vi "MainPicMotV1.vi"() -> ()   [LabVIEW 2010]
uses:
  <vilib>/Instr/_visa.llb/VISA Flush IO Buffer Mask.ctl
  Variable globale 1.vi
  <vilib>/Instr/_visa.llb/VISA Configure Serial Port (Instr).vi
panel:
  out "Iteration 3":i32
  out "Iteration reception":i32
  out "Iteration Envoi":i32
  out "Checksum calculé":i32
  out "Checksum reçu":i32
  out "Data":i32
  out "Type de donnee (ID)":i32
  out "Byte Start ?":bool
  out "Retour 2":string
  in  "Donnee":i32=138 min=0 max=255
  in  "Type":i32=138 min=138 max=139
  in  "stop secu":bool
  in  "STOP":bool
  out "error out":errorcluster caption="sortie d'erreur"
  in  "baud rate (9600)":u32=9600 caption="débit en bauds (9600)"
  in  "Port Com":refnum<visa-resource-name> caption="Nom de ressource VISA"
  # "Envoi"
  # "Réception"
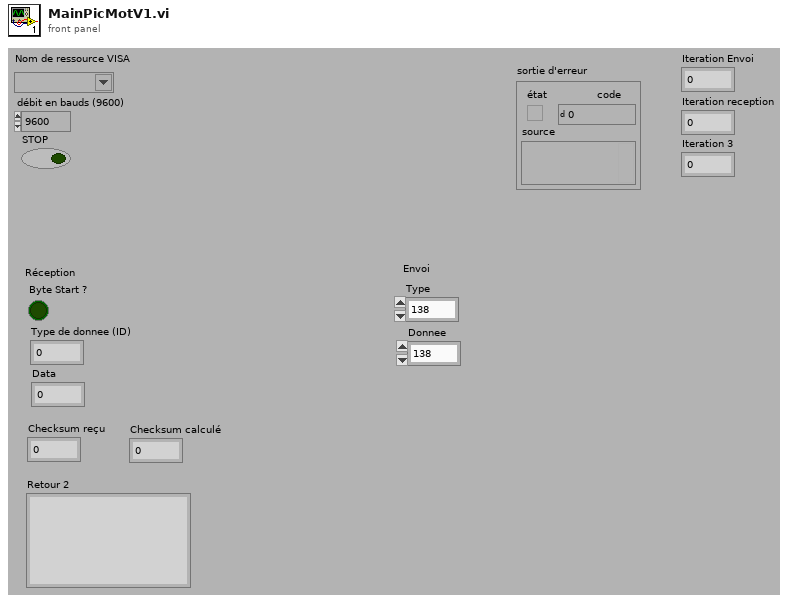
[diagram p1: front panel]
types:
  T1 = typedef "VISA Flush IO Buffer Mask.ctl" = u16
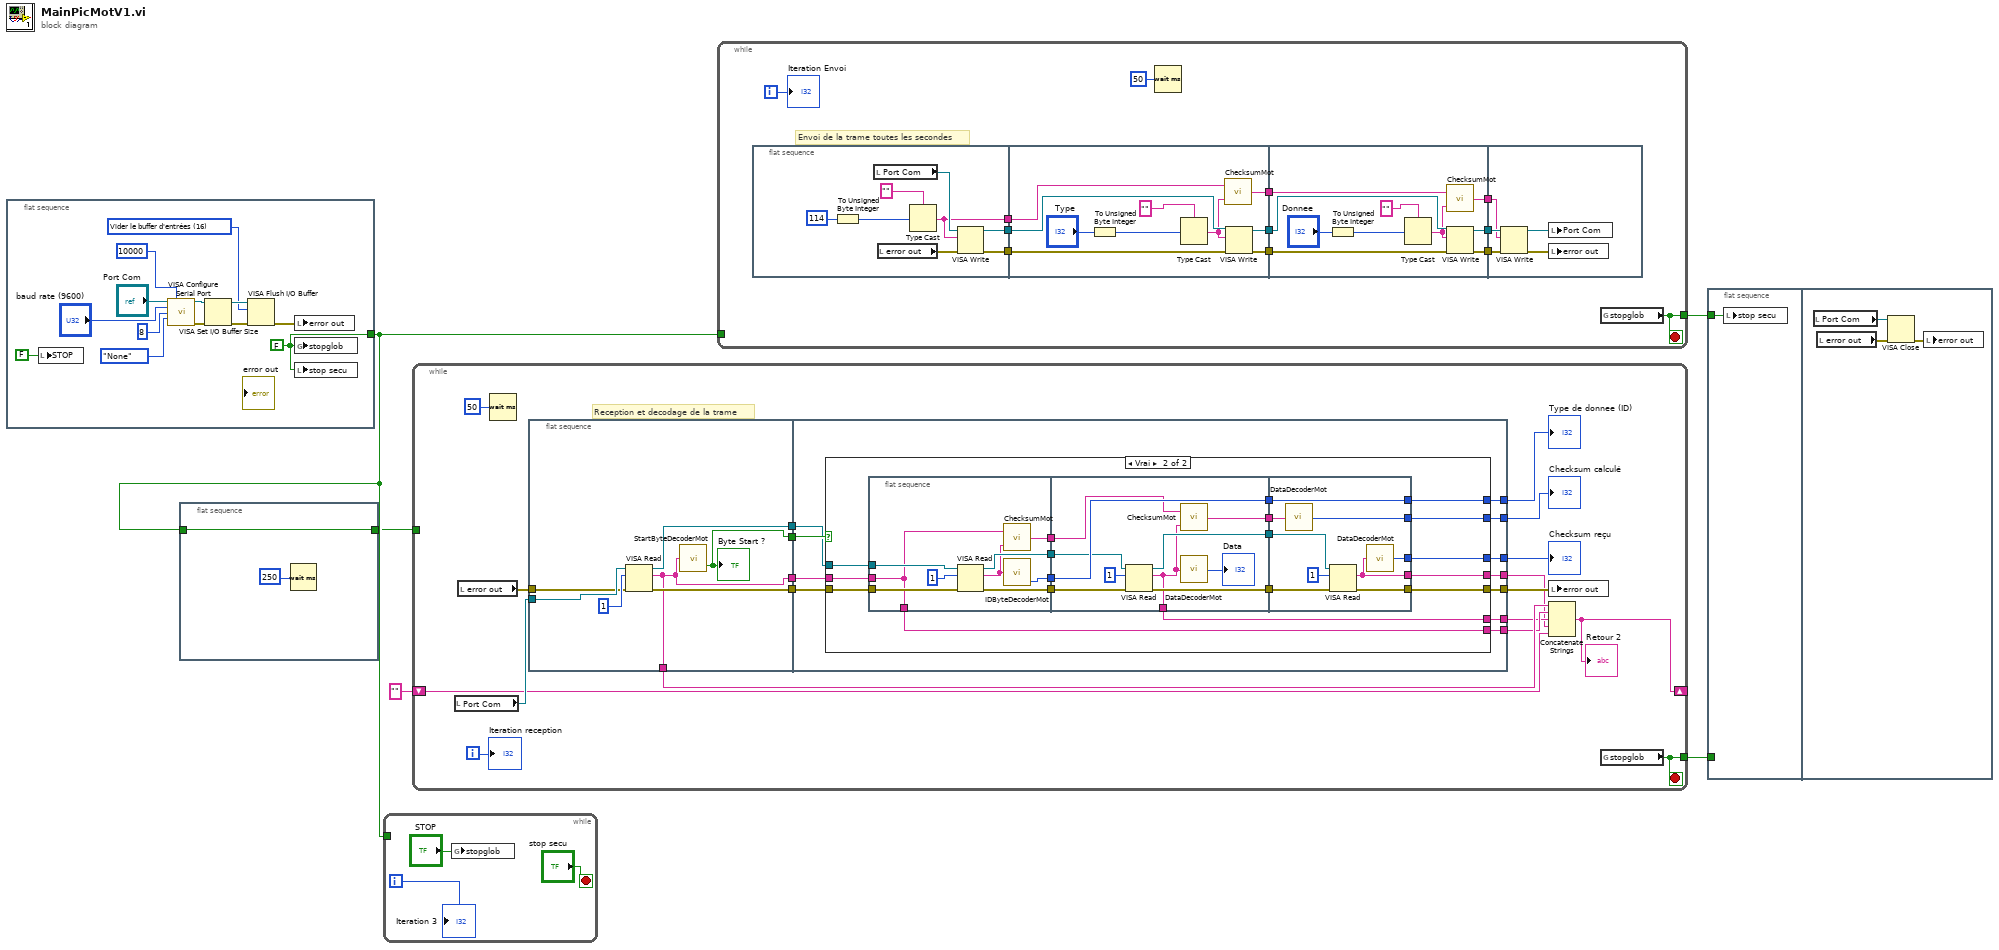
[diagram p0: block diagram]
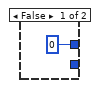
[diagram p2: hidden frame]
diagram:
  n1 = flat-sequence {
    tunnel: [w6] -> w2
    frame #0 {
      w6 = FALSE
      w9 = T1 16 items=["Vider le buffer d'entrées"=16, "Écrire le buffer de sorties sur le périphérique"=32, "Vider le buffer d'entrées (Pas d'E/S)"=64, "Vider le buffer de sorties"=128] ("Mask")
      n2 = local write "STOP"(FALSE) -> ()
      n3 = call-poly "VISA Configure Serial Port"("VISA resource name"="Port Com", "timeout (10sec)"=u32 10000, "baud rate (9600)"="baud rate (9600)", "data bits (8)"=u16 8, "parity (0:none)"=enum16{"None", "Odd", "Even", "Mark", "Space"}."None") -> ("VISA resource name out"=w13:refnum<visa-resource-name>, "error out"=w12:errorcluster)  [unwired: 9 in]
      n4 = VISA Set I/O Buffer Size(VISA resource name=w13, error in (no error)=w12) -> (VISA resource name out=w10:refnum<visa-resource-name>, error out=w11:errorcluster)  [unwired: 2 in]
      n5 = VISA Flush I/O Buffer(VISA resource name=w10, mask (16)=w9, error in (no error)=w11) -> (error out=w7:errorcluster)  [unwired: 1 out]
      n6 = local write "error out"(w7) -> ()
      n7 = global write "Variable globale 1.vi" "stopglob"(w6) -> ()
      n8 = local write "stop secu"(w6) -> ()
    }
  }
  n9 = flat-sequence {
    tunnel: w2 -> [w19]
    tunnel: [w19] -> w1
    frame #0 {
      n10 = Wait (ms)(milliseconds to wait=u32 250 ("attente (ms)")) -> ()  [unwired: 1 out]
    }
  }
  n11 = while {
    tunnel: w2 -> [_]
    i -> [w21]
    stop <- "stop secu" stop-if-true
    n12 = global write "Variable globale 1.vi" "stopglob"("STOP") -> ()
    "Iteration 3" <- w21
  }
  n13 = while {
    tunnel: [w42] -> w4
    shift-right: [w25] -> _
    shift-left: "" -> [w26]
    tunnel: w1 -> [_]
    i -> [w24]
    stop <- w42 stop-if-true
    # "Reception et decodage de la trame"
    n14 = local read "Port Com"() -> (w40:refnum<visa-resource-name>)
    n15 = local read "error out"() -> (w39:errorcluster)
    n16 = Wait (ms)(milliseconds to wait=u32 50 ("attente (ms)")) -> ()  [unwired: 1 out]
    n17 = flat-sequence {
      tunnel: w40 -> [w48]
      tunnel: w39 -> [w47]
      tunnel: [w46] -> w38
      tunnel: [w45] -> w37
      tunnel: [w44] -> w36
      tunnel: [w43] -> w34
      tunnel: [w43] -> w30
      tunnel: w38 -> [w60]
      tunnel: w37 -> [w59]
      tunnel: w36 -> [w58]
      tunnel: [w57] -> w35
      tunnel: w34 -> [w56]
      tunnel: [w55] -> w33
      tunnel: [w54] -> w32
      tunnel: [w53] -> w31
      tunnel: [w52] -> w29
      tunnel: [w51] -> w28
      tunnel: [w50] -> w27
      frame #0 {
        n18 = VISA Read(VISA resource name=w48, byte count=u32 1 ("nombre d'octets"), error in (no error)=w47) -> (VISA resource name out=w45:refnum<visa-resource-name>, read buffer=w43:string, error out=w44:errorcluster)  [unwired: 1 out]
        n19 = call "StartByteDecoderMot.vi"("byte1"=w43) -> ("Byte Start ?"=w46:bool)  [unwired: 1 in]
        "Byte Start ?" <- w46
      }
      frame #1 {
        n20 = case shown="Vrai" w60 {
          tunnel: w59 -> [_ w79]
          tunnel: w58 -> [_ w78]
          tunnel: [0 ("Type de donnee (ID)") w77] -> w57
          tunnel: w56 -> [_ w70]
          tunnel: [_ w67] -> w55
          tunnel: [_ w66] -> w54
          tunnel: [_ w65] -> w53
          tunnel: [_ w64] -> w52
          tunnel: [_ w63] -> w51
          tunnel: [_ w62] -> w50
          frame False {
          }
          frame True {
            n21 = flat-sequence {
              tunnel: w79 -> [w88]
              tunnel: w78 -> [w87]
              tunnel: [w85] -> w76
              tunnel: [w84] -> w75
              tunnel: [w83] -> w74
              tunnel: w70 -> [w80]
              tunnel: [w81] -> w69
              tunnel: [w80] -> w64
              tunnel: w76 -> [w98]
              tunnel: w75 -> [w97]
              tunnel: w74 -> [w96]
              tunnel: [w98] -> w73
              tunnel: [w93] -> w72
              tunnel: [w92] -> w71
              tunnel: w69 -> [w91]
              tunnel: [w90] -> w68
              tunnel: [w89] -> w63
              tunnel: [w107] -> w77
              tunnel: w73 -> [w107]
              tunnel: w72 -> [w106]
              tunnel: w71 -> [w105]
              tunnel: w68 -> [w103]
              tunnel: [w102] -> w67
              tunnel: [w101] -> w66
              tunnel: [w100] -> w65
              tunnel: [w99] -> w62
              frame #0 {
                n22 = VISA Read(VISA resource name=w88, byte count=u32 1 ("nombre d'octets"), error in (no error)=w87) -> (VISA resource name out=w84:refnum<visa-resource-name>, read buffer=w82:string, error out=w83:errorcluster)  [unwired: 1 out]
                n23 = call "ChecksumMot.vi"("Byte2"=w82, "Byte1"=w80) -> ("chaîne"=w81:string)
                n24 = call "IDByteDecoderMot.vi"("byte1"=w82) -> ("Type de donnee (ID)"=w85:i32)  [unwired: 2 out]
              }
              frame #1 {
                n25 = VISA Read(VISA resource name=w97, byte count=u32 1 ("nombre d'octets"), error in (no error)=w96) -> (VISA resource name out=w93:refnum<visa-resource-name>, read buffer=w89:string, error out=w92:errorcluster)  [unwired: 1 out]
                n26 = call "ChecksumMot.vi"("Byte2"=w89, "Byte1"=w91) -> ("chaîne"=w90:string)
                n27 = call "DataDecoderMot.vi"("byte1"=w89) -> ("Data"=→"Data":i32)
              }
              frame #2 {
                n28 = call "DataDecoderMot.vi"("byte1"=w103) -> ("Data"=w102:i32)
                n29 = VISA Read(VISA resource name=w106, byte count=u32 1 ("nombre d'octets"), error in (no error)=w105) -> (read buffer=w99:string, error out=w100:errorcluster)  [unwired: 2 out]
                n30 = call "DataDecoderMot.vi"("byte1"=w99) -> ("Data"=w101:i32)
              }
            }
          }
        }
      }
    }
    n31 = local write "error out"(w31) -> ()
    n32 = Concatenate Strings(w30, w29, w28, w27, w26) -> (w25:string)
    "Retour 2" <- w25
    n33 = global read "Variable globale 1.vi" "stopglob"() -> (w42:bool)
    "Type de donnee (ID)" <- w35
    "Checksum reçu" <- w32
    "Checksum calculé" <- w33
    "Iteration reception" <- w24
  }
  n34 = while {
    tunnel: [w110] -> w5
    tunnel: w2 -> [_]
    i -> [w109]
    stop <- w110 stop-if-true
    # "Envoi de la trame toutes les secondes"
    n35 = flat-sequence {
      tunnel: [w123] -> w119
      tunnel: [w122] -> w118
      tunnel: [w121] -> w113
      tunnel: w119 -> [w135]
      tunnel: w118 -> [w134]
      tunnel: [w133] -> w117
      tunnel: [w132] -> w116
      tunnel: w113 -> [w131]
      tunnel: [w129] -> w112
      tunnel: w117 -> [w147]
      tunnel: w116 -> [w146]
      tunnel: [w143] -> w115
      tunnel: [w142] -> w114
      tunnel: w112 -> [w141]
      tunnel: [w139] -> w111
      tunnel: w115 -> [w152]
      tunnel: w114 -> [w151]
      tunnel: w111 -> [w150]
      frame #0 {
        n36 = To Unsigned Byte Integer(number=114) -> (unsigned 8bit integer=w120:u8)
        n37 = local read "Port Com"() -> (w127:refnum<visa-resource-name>)
        n38 = local read "error out"() -> (w124:errorcluster)
        n39 = Type Cast(type="", x=w120) -> (*(type *) &x=w121:string)
        n40 = VISA Write(VISA resource name=w127, write buffer=w121, error in (no error)=w124) -> (VISA resource name out=w123:refnum<visa-resource-name>, error out=w122:errorcluster)  [unwired: 1 out]
      }
      frame #1 {
        n41 = To Unsigned Byte Integer(number="Type") -> (unsigned 8bit integer=w128:u8)
        n42 = Type Cast(type="", x=w128) -> (*(type *) &x=w130:string)
        n43 = call "ChecksumMot.vi"("Byte2"=w130, "Byte1"=w131) -> ("chaîne"=w129:string)
        n44 = VISA Write(VISA resource name=w135, write buffer=w130, error in (no error)=w134) -> (VISA resource name out=w132:refnum<visa-resource-name>, error out=w133:errorcluster)  [unwired: 1 out]
      }
      frame #2 {
        n45 = To Unsigned Byte Integer(number="Donnee") -> (unsigned 8bit integer=w138:u8)
        n46 = Type Cast(type="", x=w138) -> (*(type *) &x=w140:string)
        n47 = call "ChecksumMot.vi"("Byte2"=w140, "Byte1"=w141) -> ("chaîne"=w139:string)
        n48 = VISA Write(VISA resource name=w146, write buffer=w140, error in (no error)=w147) -> (VISA resource name out=w142:refnum<visa-resource-name>, error out=w143:errorcluster)  [unwired: 1 out]
      }
      frame #3 {
        n49 = VISA Write(VISA resource name=w151, write buffer=w150, error in (no error)=w152) -> (VISA resource name out=w149:refnum<visa-resource-name>, error out=w148:errorcluster)  [unwired: 1 out]
        n50 = local write "Port Com"(w149) -> ()
        n51 = local write "error out"(w148) -> ()
      }
    }
    n52 = Wait (ms)(milliseconds to wait=u32 50 ("attente (ms)")) -> ()  [unwired: 1 out]
    n53 = global read "Variable globale 1.vi" "stopglob"() -> (w110:bool)
    "Iteration Envoi" <- w109
  }
  n54 = flat-sequence {
    tunnel: w5 -> [w153]
    tunnel: w4 -> [_]
    frame #0 {
      n55 = local write "stop secu"(w153) -> ()
    }
    frame #1 {
      n56 = local read "Port Com"() -> (w156:refnum<visa-resource-name>)
      n57 = local read "error out"() -> (w155:errorcluster)
      n58 = VISA Close(VISA resource name=w156, error in (no error)=w155) -> (error out=w154:errorcluster)
      n59 = local write "error out"(w154) -> ()
    }
  }
